vi "Save_Raw_data.vi"(0 "LDA Binary":u16[][](array[numeric]), 1 "Block Timings":T1={"Started"=0.0, "Ended"=0.0, "Analogue Frequency Hz"=1000.0} {"Analogue Frequency Hz" format="%.2f"}, 2 "append to file? (new file:F)":bool, 3 "Analogue Binary":i16[][](array[numeric]), 4 "PWA Binary":i16[][](array[numeric])) -> (5 "Block Header":string)   [LabVIEW 2010]
uses:
  Controls/Block_start_and_end.ctl
  Globals/Constants_global.vi
  Globals/Meas_global.vi
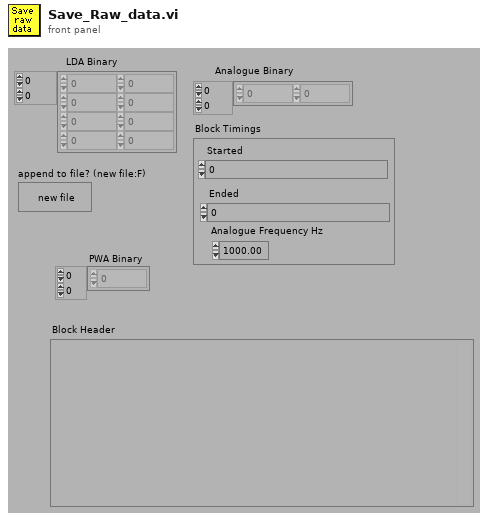
[diagram p1: front panel]
types:
  T1 = typedef "Block_start_and_end.ctl" = cluster{"Started":dbl, "Ended":dbl, "Analogue Frequency Hz":dbl}
  T2 = typedef "PWA_Data.ctl" = enum16{"No PWA Data", "One Ch PWA"}
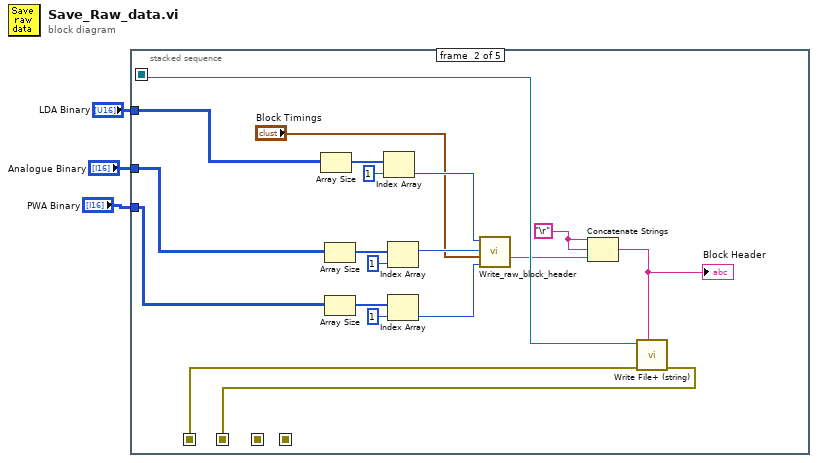
[diagram p0: block diagram]
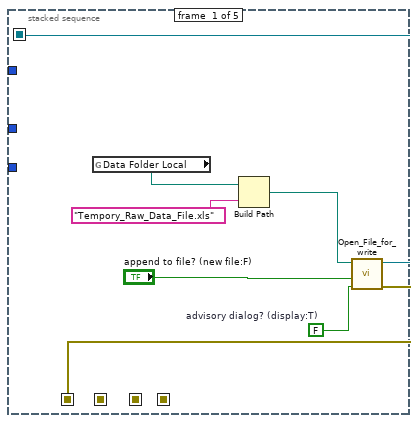
[diagram p2: hidden frame]
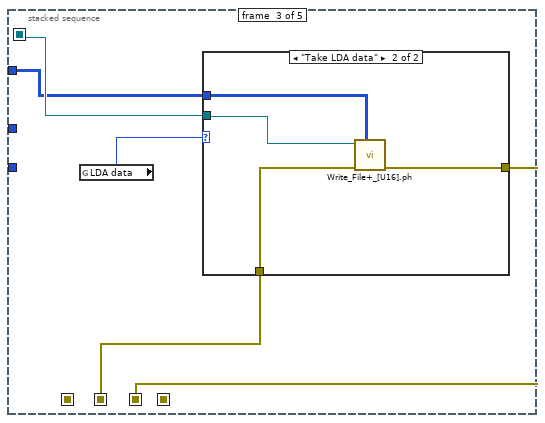
[diagram p3: hidden frame]
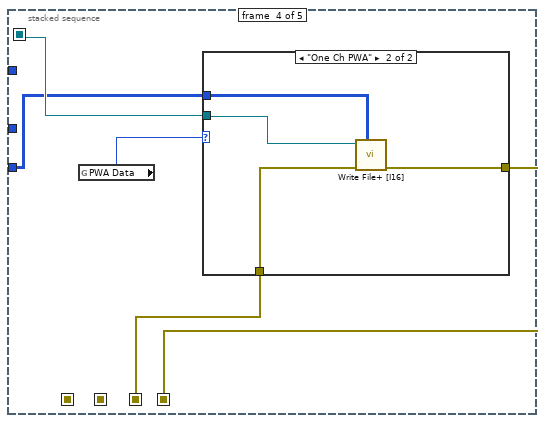
[diagram p5: hidden frame]
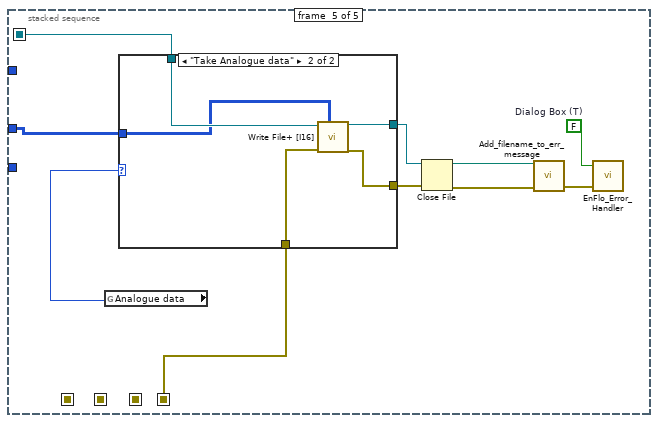
[diagram p7: hidden frame]
diagram:
  n1 = stacked-sequence {
    seq-local: [w10 _ _ _ _] -> [_ w23 w33 w43 w58]
    seq-local: [w9 _ _ _ _] -> [_ w22 _ _ _]
    seq-local: [_ w21 _ _ _] -> [_ _ w32 _ _]
    seq-local: [_ _ w31 _ _] -> [_ _ _ w42 _]
    seq-local: [_ _ _ w41 _] -> [_ _ _ _ w50]
    tunnel: "LDA Binary" -> [_ w17 w30 _ _]
    tunnel: "Analogue Binary" -> [_ w16 _ _ w51]
    tunnel: "PWA Binary" -> [_ w13 _ w40 _]
    frame #0 {
      w8 = FALSE  # advisory dialog? (display:T)
      n2 = global read "Constants_global.vi" "Data Folder Local"() -> (w7:path)
      n3 = Build Path(base path=w7, name or relative path="Tempory_Raw_Data_File.xls") -> (appended path=w5:path)
      n4 = call "Open_File_for_write.vi"("advisory dialog? (display:T)"=w8, "append to file? (new file:F)"="append to file? (new file:F)", "file path"=w5) -> ("error out"=w9:errorcluster, "refnum"=w10:refnum<file>)  [unwired: 7 out]
    }
    frame #1 {
      w18 = "\r"
      n5 = Array Size(array=w17) -> (size(s)=w28:i32[])
      n6 = Array Size(array=w16) -> (size(s)=w27:i32[])
      n7 = Array Size(array=w13) -> (size(s)=w14:i32[])
      n8 = Index Array(array=w28, index=1) -> (element=w25:i32)
      n9 = Index Array(array=w27, index=1) -> (element=w24:i32)
      n10 = Index Array(array=w14, index=1) -> (element=w12:i32)
      n11 = call "Write_raw_block_header.vi"("No of PWA samples"=w12, "Block Timings"="Block Timings", "No of analogue samples"=w24, "No of LDA samples"=w25) -> ("Output string"=w19:string)
      n12 = Concatenate Strings(w18, w18, w19) -> (w11:string)
      "Block Header" <- w11
      n13 = call <vilib>:"Write File+ (string).vi"("string"=w11, "error in (no error)"=w22, "refnum"=w23) -> ("error out"=w21:errorcluster)  [unwired: 2 in, 4 out]
    }
    frame #2 {
      n14 = global read "Meas_global.vi" "LDA data"() -> (w34:enum16{"No LDA data", "Take LDA data"})
      n15 = case shown="\"Take LDA data\"" w34 {
        tunnel: w30 -> [_ w39]
        tunnel: w33 -> [_ w38]
        tunnel: w32 -> [w35 w37]
        tunnel: [w35 w36] -> w31
        frame "No LDA data" {
        }
        frame "Take LDA data" {
          n16 = call "Write_File+_[U16].ph.vi"("2D array"=w39, "error in (no error)"=w37, "refnum"=w38) -> ("error out"=w36:errorcluster)  [unwired: 3 in, 5 out]
        }
      }
    }
    frame #3 {
      n17 = global read "Meas_global.vi" "PWA Data"() -> (w44:T2)
      n18 = case shown="\"One Ch PWA\"" w44 {
        tunnel: w40 -> [_ w47]
        tunnel: w43 -> [_ w46]
        tunnel: w42 -> [w45 w49]
        tunnel: [w45 w48] -> w41
        frame "No PWA Data" {
        }
        frame "One Ch PWA" {
          n19 = call <vilib>:"Write File+ [I16].vi"("2D array"=w47, "error in (no error)"=w49, "refnum"=w46) -> ("error out"=w48:errorcluster)  [unwired: 3 in, 5 out]
        }
      }
    }
    frame #4 {
      w56 = FALSE  # Dialog Box (T)
      n20 = global read "Meas_global.vi" "Analogue data"() -> (w59:enum16{"No Analogue data", "Take Analogue data"})
      n21 = case shown="\"Take Analogue data\"" w59 {
        tunnel: w51 -> [_ w65]
        tunnel: w58 -> [w61 w66]
        tunnel: w50 -> [w60 w64]
        tunnel: [w60 w63] -> w55
        tunnel: [w61 w62] -> w54
        frame "No Analogue data" {
        }
        frame "Take Analogue data" {
          n22 = call <vilib>:"Write File+ [I16].vi"("2D array"=w65, "error in (no error)"=w64, "refnum"=w66) -> ("error out"=w63:errorcluster, "dup refnum"=w62:refnum<file>)  [unwired: 3 in, 4 out]
        }
      }
      n23 = Close File(refnum=w54, error in=w55) -> (path=w52:path, error out=w53:errorcluster)
      n24 = call "Add_filename_to_err_message.vi"("error in (no error)"=w53, "Path"=w52) -> ("error out"=w57:errorcluster)
      n25 = call "EnFlo_Error_Handler.vi"("error in (no error)"=w57, "Dialog Box (T)"=w56) -> ()  [unwired: 1 in, 3 out]
    }
  }
